vi "Handle Double Data.vi"(7 "Source ID":u32, 8 "GroupData":T1, 9 "Sequence":u32, 10 "ChannelService":refnum<class "ChannelService.lvclass">, 11 "Subscription Loop Data in":T2) -> (0 "error out":errorcluster, 3 "Subscription Loop Data":T2)   [LabVIEW 2020, in "Vecto.lvlib" / "RemoteDataService.lvclass"]
uses:
  RemoteDataService.lvclass
  Subscription Loop Data.ctl
  Subscription Group Info.ctl
  Group/Group.lvclass
  SubscribedDataHandler/SubscribedDataHandler.lvclass
  proto/GroupData/Data.ctl
  ChannelService/ChannelService.lvclass
  Group DBL/Group DBL.lvclass
  C:/dev/lv20CE/relink/lv-vecto/Vecto/Group/Group.lvclass
  <vilib>/Utility/miscctls.llb/LVMapReplaceAction.ctl
  Group/Group.lvclass/Group.ctl
  RemoteDataService.lvclass/RemoteDataService.ctl
  Vecto.lvlib
  proto/GroupData/GroupData.lvlib
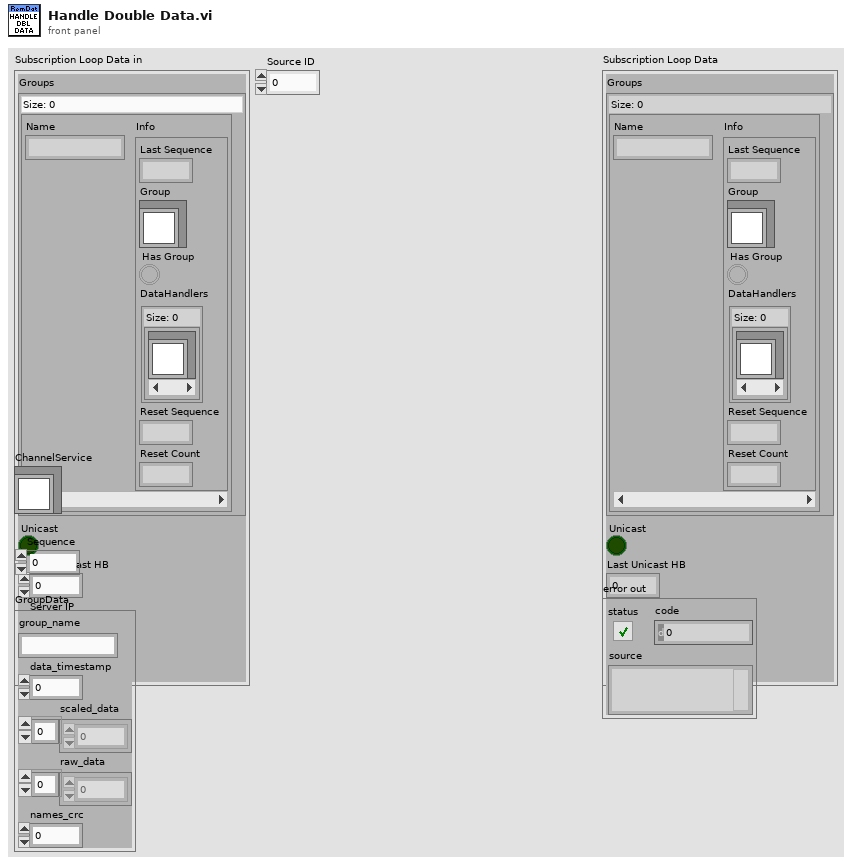
[diagram p1: front panel]
types:
  T1 = typedef "GroupData.lvlib/Data.ctl" = cluster{"group_name":string, "data_timestamp":i64, "scaled_data":dbl[], "raw_data":dbl[], "names_crc":u32}
  T2 = typedef "Vecto.lvlib/RemoteDataService.lvclass/Subscription Loop Data.ctl" = cluster{"Groups":map{string, T3}, "Unicast":bool, "Last Unicast HB":dbl, "Server IP":u32, "Server Port":u16}
  T3 = typedef "Vecto.lvlib/RemoteDataService.lvclass/Subscription Group Info.ctl" = cluster{"Last Sequence":u32, "Group":refnum<class "Group.lvclass">, "Has Group":bool, "DataHandlers":set{refnum<class "SubscribedDataHandler.lvclass">}, "Reset Sequence":u32, "Reset Count":u32}
  T4 = typedef "LVMapReplaceAction.ctl" = enum32{"Modify Entry only if found", "Add or Modify Entry", "Delete Entry"}
  T5 = set{refnum<class "SubscribedDataHandler.lvclass">}
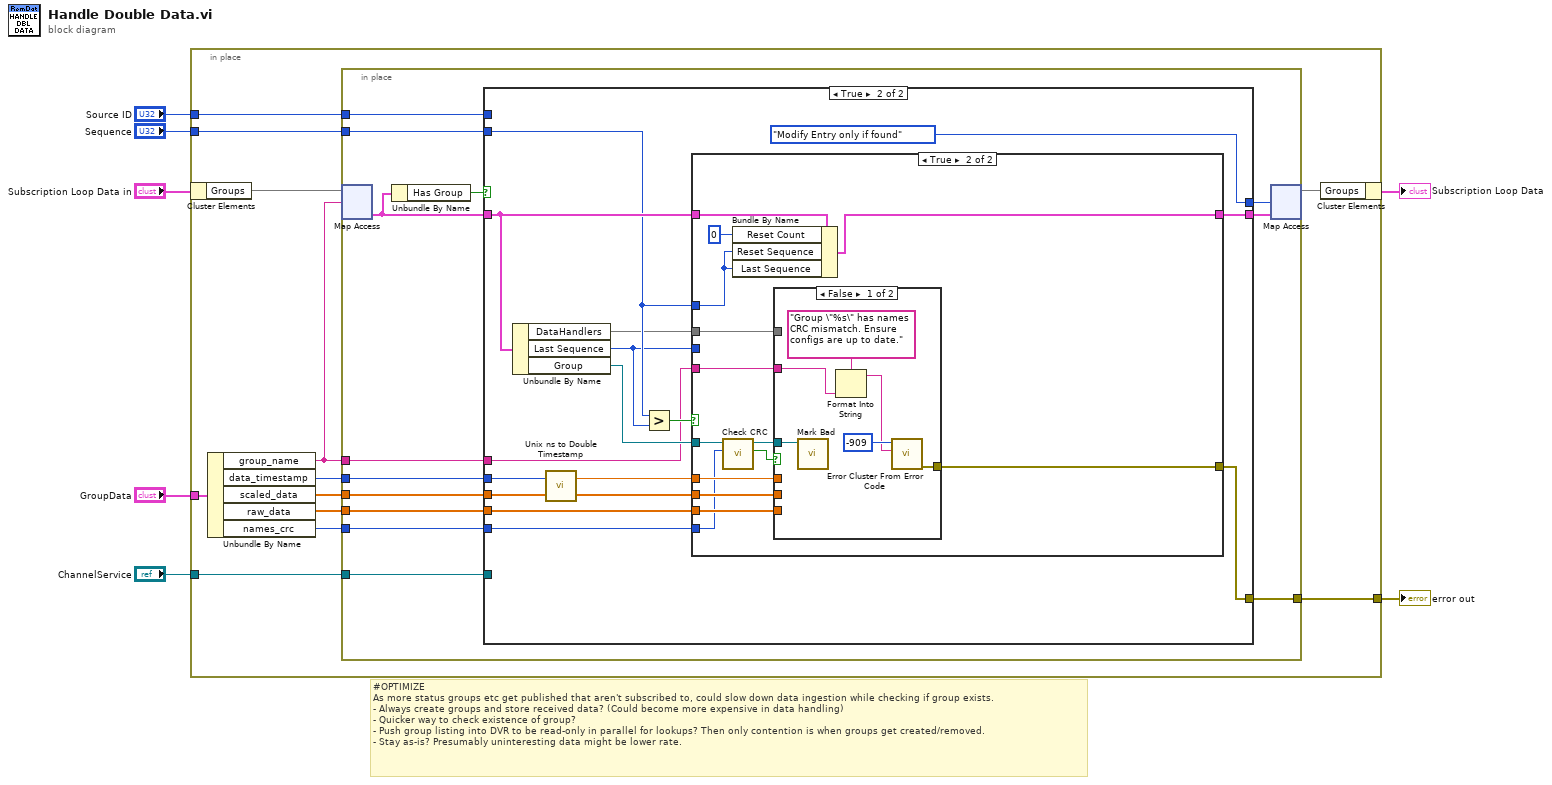
[diagram p0: block diagram]
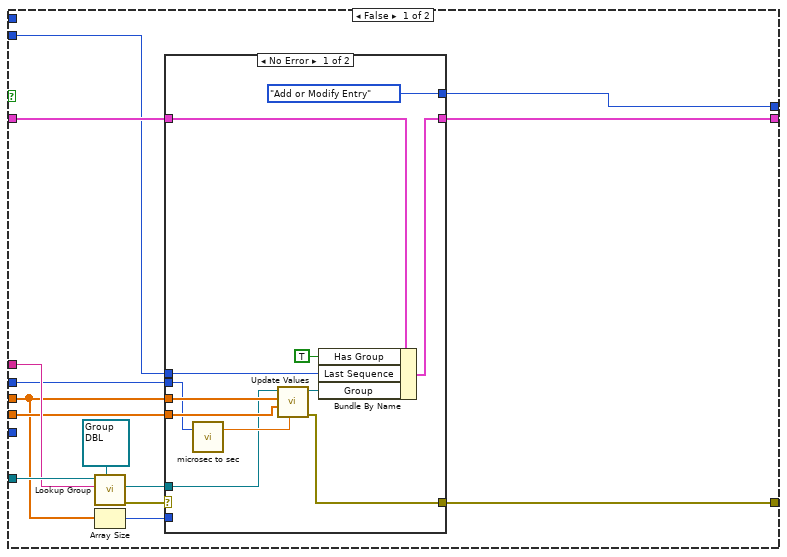
[diagram p2: hidden frame]
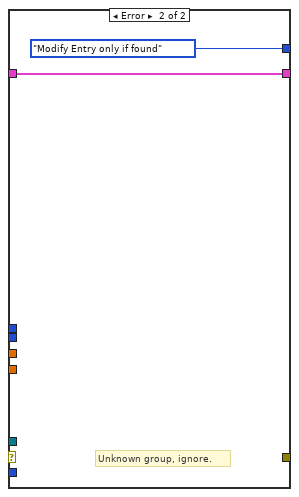
[diagram p3: hidden frame]
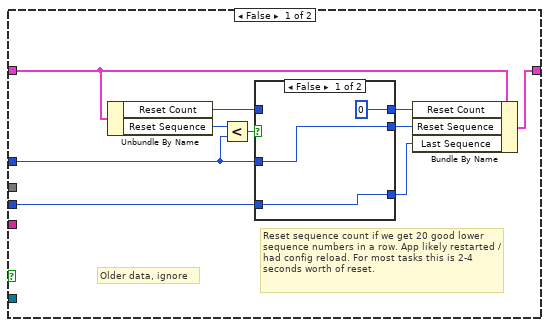
[diagram p4: hidden frame]
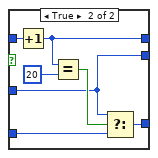
[diagram p5: hidden frame]
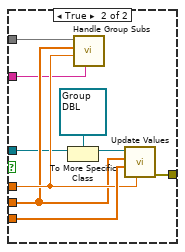
[diagram p6: hidden frame]
diagram:
  # "#OPTIMIZE\nAs more status groups etc get published that aren't subscribed to, could slow down data ingestion while checking if group exists.\n- Always create groups and store received data? (Could become more expensive in data handling)\n- Quicker way to check existence of group?\n- Push group listing into DVR to be read-only in parallel for lookups? Then only contention is when groups get created/removed.\n- Stay as-is? Presumably uninteresting data might be lower rate."
  n1 = in-place {
    in-place-border: "GroupData" -> [w10]
    in-place-border: "ChannelService" -> [w18]
    in-place-border: "Sequence" -> [w14]
    in-place-border: "Source ID" -> [w13]
    in-place-border: [w11] -> w2
    n2 = in-place-cluster #1("Subscription Loop Data in") -> ("Groups"=w19:map{string, T3})
    n3 = Unbundle By Name(w10) -> ("group_name"=w8:string, "data_timestamp"=w15:i64, "scaled_data"=w16:dbl[], "raw_data"=w17:dbl[], "names_crc"=w9:u32)
    n4 = in-place {
      in-place-border: w18 -> [w32]
      in-place-border: w8 -> [w31]
      in-place-border: w17 -> [w30]
      in-place-border: w16 -> [w29]
      in-place-border: w15 -> [w28]
      in-place-border: w14 -> [w27]
      in-place-border: w13 -> [w26]
      in-place-border: [w24] -> w11
      in-place-border: w9 -> [w20]
      n5 = in-place-map #2(w19, w8) -> (w22:T3)  [unwired: 1 in, 1 out]
      n6 = Unbundle By Name(w22) -> ("Has Group"=w21:bool)
      n7 = case shown="True" w21 {
        tunnel: w22 -> [w41 w70]
        tunnel: w32 -> [w46 _]
        tunnel: w31 -> [w44 w64]
        tunnel: w30 -> [w39 w71]
        tunnel: w29 -> [w38 w72]
        tunnel: w28 -> [w33 w73]
        tunnel: w27 -> [w40 w68]
        tunnel: w26 -> [_ _]
        tunnel: [w37 w69] -> w25
        tunnel: [w36 w67] -> w24
        tunnel: [w35 LVMapReplaceAction."Modify Entry only if found" ("action")] -> w23
        tunnel: w20 -> [_ w61]
        frame False {
          n8 = call "Lookup Group.vi"("Group Type (Abstract)"=refnum<class "Group DBL.lvclass"> refnum ("Vecto.lvlib:Group.lvclass"), "Group Name"=w44, "ChannelService in"=w46) -> ("error out"=w45:errorcluster, "Group"=w43:refnum<class "Group DBL.lvclass">)  [unwired: 6 in, 1 out]
          n9 = Array Size(array=w38) -> (size(s)=w42:i32)
          n10 = case shown="No Error" w45 {
            tunnel: w43 -> [w49 _]
            tunnel: w42 -> [_ _]
            tunnel: w41 -> [w48 w59]
            tunnel: w40 -> [w58 _]
            tunnel: w39 -> [w57 _]
            tunnel: w38 -> [w56 _]
            tunnel: [w55 w59] -> w37
            tunnel: [w54 _] -> w36
            tunnel: [LVMapReplaceAction."Add or Modify Entry" ("action") LVMapReplaceAction."Modify Entry only if found" ("action")] -> w35
            tunnel: w33 -> [w51 _]
            frame No Error {
              n11 = call "microsec to sec.vi"("data_timestamp us"=w51) -> ("timestamp s"=w50:dbl)  [unwired: 2 in]
              n12 = call "Update Values.vi"("Timestamp (Now)"=w50, "Raw Values (N/A)"=w57, "Values"=w56, "Group in"=w49) -> ("error out"=w54:errorcluster, "Group out"=w53:refnum<class "Group DBL.lvclass">)  [unwired: 6 in]
              n13 = Bundle By Name(cluster=w48, "Has Group"=TRUE, "Last Sequence"=w58, "Group"=w53) -> (w55:T3)
            }
            frame Error {
              # "Unknown group, ignore."
            }
          }
        }
        frame True {
          n14 = Unbundle By Name(w70) -> ("DataHandlers"=w63:T5, "Last Sequence"=w62:u32, "Group"=w75:refnum<class "Group.lvclass">)
          n15 = call "Unix ns to Double Timestamp.vi"("unix ns"=w73) -> ("Timestamp"=w65:dbl)  [unwired: 2 in]
          n16 = Greater?(x=w68, y=w62) -> (0:w74:bool)
          n17 = case shown="True" w74 {
            tunnel: w75 -> [_ w109]
            tunnel: w65 -> [_ w104]
            tunnel: w72 -> [_ w103]
            tunnel: w71 -> [_ w108]
            tunnel: w70 -> [w81 w107]
            tunnel: [w79 w106] -> w69
            tunnel: w68 -> [w82 w100]
            tunnel: [_ w105] -> w67
            tunnel: w64 -> [_ w102]
            tunnel: w63 -> [_ w101]
            tunnel: w62 -> [w83 _]
            tunnel: w61 -> [_ w97]
            frame False {
              # "Reset sequence count if we get 20 good lower sequence numbers in a row. App likely restarted / had config reload. For most tasks this is 2-4 seconds worth of reset."
              # "Older data, ignore"
              n18 = Unbundle By Name(w81) -> ("Reset Count"=w84:u32, "Reset Sequence"=w77:u32)
              n19 = Less?(x=w77, y=w82) -> (x < y?=w85:bool)
              n20 = case shown="False" w85 {
                tunnel: w84 -> [_ w95]
                tunnel: w83 -> [w87 w93]
                tunnel: w82 -> [w86 w89]
                tunnel: [w87 w91] -> w78
                tunnel: [u32 0 w90] -> w80
                tunnel: [w86 w89] -> w76
                frame False {
                }
                frame True {
                  n21 = Increment(x=w95) -> (x+1=w90:u32)
                  n22 = Equal?(x=w90, y=u32 20) -> (x = y?=w92:bool)
                  n23 = Select(t=w89, s=w92, f=w93) -> (s? t:f=w91:u32)
                }
              }
              n24 = Bundle By Name(cluster=w81, "Reset Count"=w80, "Reset Sequence"=w76, "Last Sequence"=w78) -> (w79:T3)
            }
            frame True {
              n25 = call "Check CRC.vi"("Msg Names CRC"=w97, "Group in"=w109) -> ("CRC Matches"=w96:bool, "Group out"=w98:refnum<class "Group.lvclass">)  [unwired: 8 in]
              n26 = Bundle By Name(cluster=w107, "Reset Count"=u32 0, "Reset Sequence"=w100, "Last Sequence"=w100) -> (w106:T3)
              n27 = case shown="False" w96 {
                tunnel: w108 -> [_ w124]
                tunnel: [w114 w123] -> w105
                tunnel: w104 -> [_ w120]
                tunnel: w103 -> [_ w119]
                tunnel: w102 -> [w112 w118]
                tunnel: w101 -> [_ w117]
                tunnel: w98 -> [w115 w116]
                frame False {
                  n28 = call "Mark Bad.vi"("Group in"=w115) -> ()  [unwired: 9 in, 2 out]
                  n29 = Format Into String(format string="Group \"%s\" has names CRC mismatch. Ensure configs are up to date.", w112) -> (resulting string=w110:string)  [unwired: 2 in, 1 out]
                  n30 = call <vilib>:"Error Cluster From Error Code.vi"("error message (\"\")"=w110, "error code (0)"=-909) -> ("error out"=w114:errorcluster)  [unwired: 7 in]
                }
                frame True {
                  n31 = To More Specific Class(target class=refnum<class "Group DBL.lvclass"> refnum ("Group in"), reference=w116) -> (specific class reference=w122:refnum<class "Group DBL.lvclass">)  [unwired: 1 in, 1 out]
                  n32 = call "Handle Group Subs.vi"("Group"=w118, "Timestamp"=w120, "Data"=w119, "Data Handlers"=w117) -> ()  [unwired: 8 in]
                  n33 = call "Update Values.vi"("Timestamp (Now)"=w120, "Raw Values (N/A)"=w124, "Values"=w119, "Group in"=w122) -> ("error out"=w123:errorcluster)  [unwired: 6 in, 1 out]
                }
              }
            }
          }
        }
      }
      n34 = in-place-map #2(w25, w23) -> (w12:map{string, T3})  [unwired: 2 out]
    }
    n35 = in-place-cluster #1("Groups"=w12) -> (→"Subscription Loop Data":T2)
  }
  "error out" <- w2
